vi "Digitallypython.vi"() -> ()   [LabVIEW 2019]
panel:
  out "Array":dbl[](array[numeric])
  out "Numeric 2":dbl
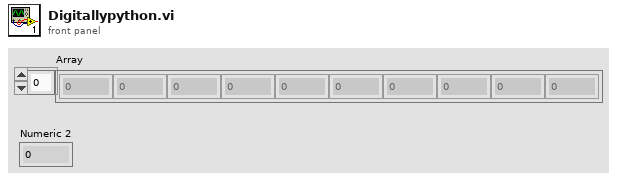
[diagram p1: front panel]
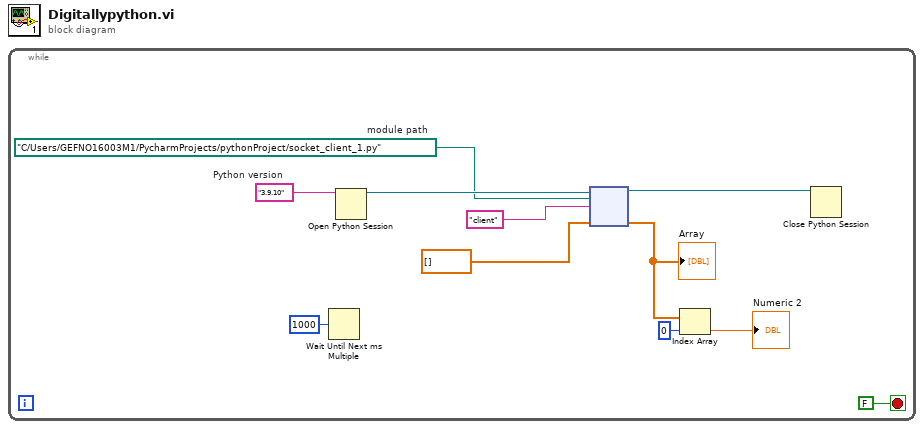
[diagram p0: block diagram]
diagram:
  n1 = while {
    stop <- FALSE stop-if-true
    w9 = path "C:/Users/GEFNO16003M1/PycharmProjects/pythonProject/socket_client_1.py"  # module path
    w11 = "3.9.10"  # Python version
    n2 = Wait Until Next ms Multiple(millisecond multiple=u32 1000) -> ()  [unwired: 1 out]
    n3 = Open Python Session(python version=w11) -> (session out=w10:refnum<k35>)  [unwired: 2 in, 1 out]
    n4 = node ("Python Node")(w10, w9, "client" ("function name"), dbl[] []) -> (w8:refnum<k35>, w6:dbl[])  [unwired: 1 in, 3 out]
    "Array" <- w6
    n5 = Index Array(array=w6, index=0) -> (element=→"Numeric 2":dbl)
    n6 = Close Python Session(session in=w8) -> ()  [unwired: 1 in, 1 out]
  }
